vi "ObjectHandler.Init.vi"(8 "error in (no error)":errorcluster, 11 "ObjectHandler in":refnum<class "ObjectHandler.lvclass">) -> (0 "error out":errorcluster, 3 "ObjectHandler out":refnum<class "ObjectHandler.lvclass">)   [LabVIEW 2016, in "ObjectHandler.lvclass"]
uses:
  ObjectHandler.lvclass
  ObjectHandler.lvclass/ObjectHandler.ctl
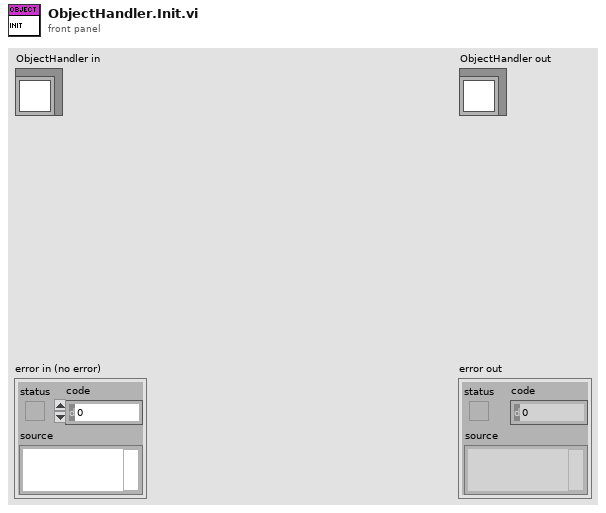
[diagram p1: front panel]
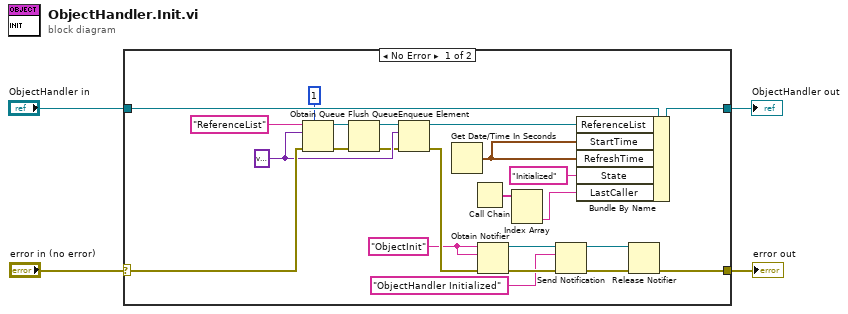
[diagram p0: block diagram]
diagram:
  n1 = case shown="No Error" "error in (no error)" {
    selector: "error in (no error)" -> [w20 w29]
    tunnel: [w9 w29] -> w3
    tunnel: [w27 w28] -> w1
    tunnel: "ObjectHandler in" -> [w26 w28]
    frame No Error {
      w5 = "ObjectInit" ("name (unnamed)")
      w18 = variant
      n2 = Obtain Queue(max queue size (-1, unlimited)=1, name (unnamed)="ReferenceList" ("Name"), element data type=w18, error in (no error)=w20) -> (queue out=w13:refnum<queue>, error out=w16:errorcluster)  [unwired: 1 in, 1 out]
      n3 = Flush Queue(queue=w13, error in (no error)=w16) -> (queue out=w14:refnum<queue>, error out=w15:errorcluster)  [unwired: 1 out]
      n4 = Enqueue Element(queue=w14, element=w18, error in (no error)=w15) -> (queue out=w19:refnum<queue>, error out=w12:errorcluster)  [unwired: 1 in, 1 out]
      n5 = Get Date/Time In Seconds() -> (seconds since 1Jan1904=w25:timestamp)
      n6 = Call Chain() -> (call chain=w23:string[])
      n7 = Obtain Notifier(name (unnamed)=w5, notification data type=w5, error in (no error)=w12) -> (notifier out=w7:refnum<notifier>, error out=w11:errorcluster)  [unwired: 1 in, 1 out]
      n8 = Index Array(array=w23) -> (element #2=w22:string)  [unwired: 2 in, 1 out]
      n9 = Send Notification(notification="ObjectHandler Initialized", notifier=w7, error in (no error)=w11) -> (notifier out=w8:refnum<notifier>, error out=w10:errorcluster)
      n10 = Bundle By Name(cluster=w26, "ReferenceList"=w19, "StartTime"=w25, "RefreshTime"=w25, "State"="Initialized", "LastCaller"=w22) -> (w27:refnum<class "ObjectHandler.lvclass">)
      n11 = Release Notifier(notifier=w8, error in (no error)=w10) -> (error out=w9:errorcluster)  [unwired: 1 in, 2 out]
    }
    frame Error {
    }
  }
  "error out" <- w3
  "ObjectHandler out" <- w1
